vi "Convert_String_to_TimeStamp2.vi"(1 "date/time string":string) -> (0 "Resulting Time Stamp":timestamp)   [LabVIEW 2013]
doc: "This VI convert a date/time string back to a time stamp."
panel:
  # "This control should have data in the form:\n4/30/2004 7:48:47 PM"
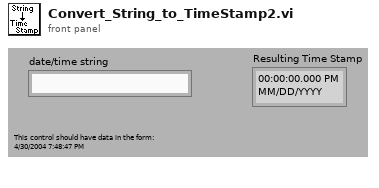
[diagram p1: front panel]
types:
  T1 = cluster{"second":i32, "minute":i32, "hour":i32, "day of month":i32, "month":i32, "year":i32, "day of week":i32, "day of year":i32, "is DST":i32}
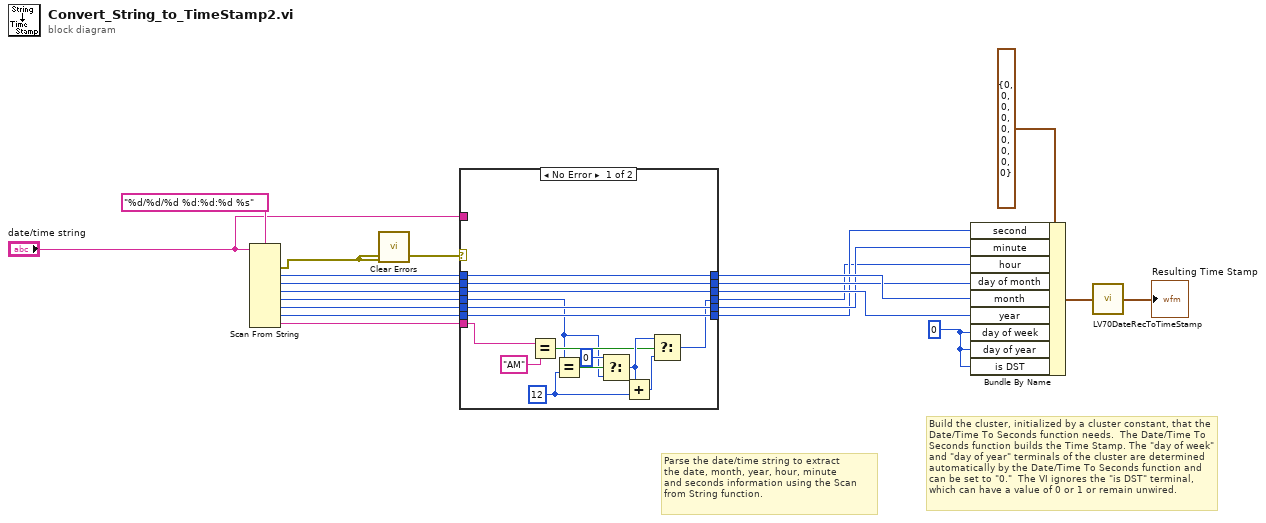
[diagram p0: block diagram]
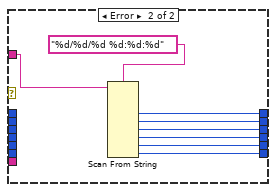
[diagram p2: hidden frame]
diagram:
  w16 = 0
  # "Build the cluster, initialized by a cluster constant, that the Date/Time To Seconds function needs.  The Date/Time To Seconds function builds the Time Stamp. The \"day of week\" and \"day of year\" terminals of the cluster are determined automatically by the Date/Time To Seconds function and can be set to \"0.\"  The VI ignores the \"is DST\" terminal, which can have a value of 0 or 1 or remain unwired."
  # "Parse the date/time string to extract \nthe date, month, year, hour, minute \nand seconds information using the Scan\nfrom String function."
  n1 = Scan From String "Scan From String"(format string="%d/%d/%d %d:%d:%d %s", input string="date/time string") -> (error out=w15:errorcluster, output 1=w14:i32, output 2=w12:i32, output 3=w10:i32, output 4=w8:i32, output 5=w7:i32, output 6=w5:i32, output 7=w3:string)  [unwired: 9 in, 2 out]
  n2 = call <vilib>:"Clear Errors.vi"("error in (no error)"=w15) -> ()  [unwired: 6 in, 1 out]
  n3 = case shown="No Error" w15 {
    tunnel: w14 -> [w35 _]
    tunnel: [w35 w41] -> w13
    tunnel: w12 -> [w34 _]
    tunnel: [w34 w40] -> w11
    tunnel: w10 -> [w33 _]
    tunnel: [w33 w39] -> w9
    tunnel: w8 -> [w22 _]
    tunnel: [w21 w38] -> w1
    tunnel: w7 -> [w32 _]
    tunnel: [w32 w37] -> w6
    tunnel: w5 -> [w31 _]
    tunnel: [w31 w36] -> w4
    tunnel: w3 -> [w23 _]
    tunnel: "date/time string" -> [_ w43]
    frame No Error {
      w27 = 12 ("y")
      n4 = Equal?(x=w23, y="AM") -> (x = y?=w26:bool)
      n5 = Equal?(x=w22, y=w27) -> (x = y?=w28:bool)
      n6 = Select(t=0, s=w28, f=w22) -> (s? t:f=w29:i32)
      n7 = Add(x=w29, y=w27) -> (x+y=w25:i32)
      n8 = Select(t=w29, s=w26, f=w25) -> (s? t:f=w21:i32)
    }
    frame Error {
      n9 = Scan From String "Scan From String"(format string="%d/%d/%d %d:%d:%d", input string=w43) -> (output 1=w41:i32, output 2=w40:i32, output 3=w39:i32, output 4=w38:i32, output 5=w37:i32, output 6=w36:i32)  [unwired: 8 in, 3 out]
    }
  }
  n10 = Bundle By Name(cluster=T1 {"second"=0, "minute"=0, "hour"=0, "day of month"=0, "month"=0, "year"=0, "day of week"=0, "day of year"=0, "is DST"=0} ("date time rec"), "second"=w4, "minute"=w6, "hour"=w1, "day of month"=w11, "month"=w13, "year"=w9, "day of week"=w16, "day of year"=w16, "is DST"=w16) -> (w17:T1)
  n11 = call <vilib>:"LV70DateRecToTimeStamp.vi"("date time rec"=w17) -> ("Time Stamp"=→"Resulting Time Stamp":timestamp)
